vi "CheckLibraries.vi"(11 "hub":string) -> (0 "error out":errorcluster, 3 "console out":string)   [LabVIEW 2022 SP3]
panel:
  out "Array":bool[](array[boolean])
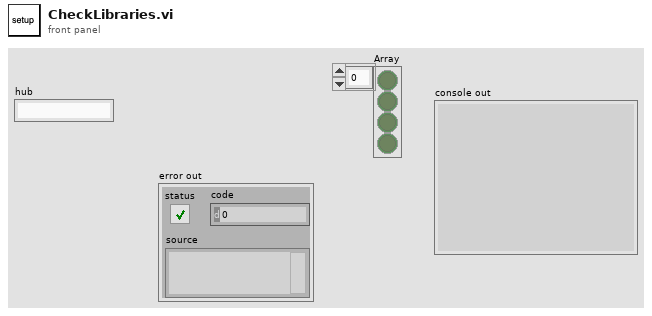
[diagram p1: front panel]
types:
  T1 = typedef "PythonCtrl.ctl" = cluster{"session":refnum<k35>, "PyPath":path, "Processor":T2, "Port":string, "version":string}
  T2 = typedef "Processors.ctl" = enum16{"SPIKE", "Pi", "Pi_ssh", "OpenMV", "Dunio"}
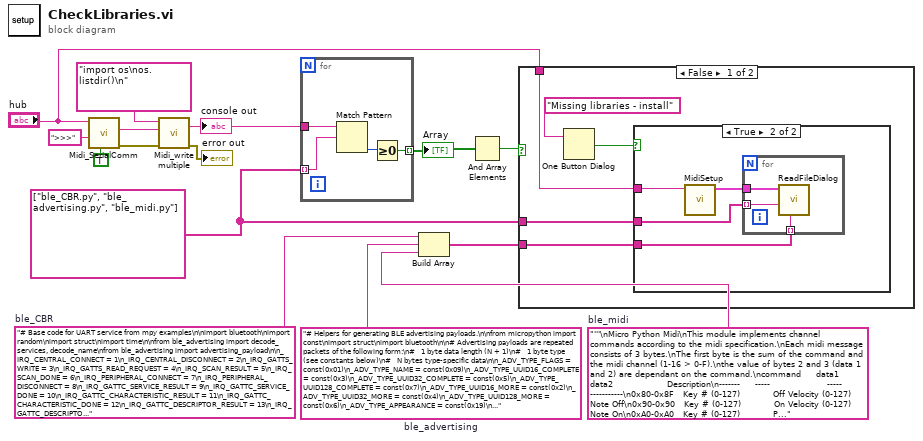
[diagram p0: block diagram]
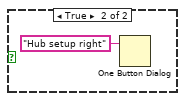
[diagram p3: hidden frame]
diagram:
  w4 = "'''\nMicro Python Midi\nThis module implements channel commands according to the midi specification.\nEach midi message consists of 3 bytes.\nThe first byte is the sum of the command and the midi channel (1-16 > 0-F).\nthe value of bytes 2 and 3 (data 1 and 2) are dependant on the command.\ncommand     data1                   data2                  Description\n-------     -----                   -----                  -----------\n0x80-0x8F   Key # (0-127)           Off Velocity (0-127)   Note Off\n0x90-0x90   Key # (0-127)           On Velocity (0-127)    Note On\n0xA0-0xA0   Key # (0-127)           Pressure (0-127)       Poly Pressure\n0xB0-0xB0   Control # (0-127)       Control Value (0-127)  Control\n0xC0-0xC0   Program # (0-127)       Not Used (send 0)      Program Change\n0xD0-0xD0   Pressure Value (0-127)  Not Used (send 0)      Channel Pressure\n0xE0-0xE0   Range LSB (0-127)       Range MSB (0-127)      Pitch Bend\nhttp://www.midi.org/techspecs/midimessages.php\n'''\n\nimport struct\nimport ble_CBR\nimport bluetooth\nimport button\nimport time\nimport distance_sensor as ds\nimport port,time\nimport color_sensor as cs\n\ndone = lambda : button.button_pressed(button.BUTTON_RIGHT)\n\npackage = [0x00,0x00,0x00,0x00,0x00]\n\nclass midi:\n    def __init__(self, name = 'MySpike'):\n        n = name[0:7]\n        self.connection = ble_CBR.BLESimplePeripheral(bluetooth.BLE(), 'MIDI', n)\n        self.connection.on_write(self.on_receive)\n        self.buffer = []\n        \n    def on_receive(self, msg):\n        print(\"RX: \", msg)\n      \n    def connected(self):\n        return self.connection.is_connected()\n\n    def convert(self, cmd, value, volume):\n        timestamp_ms = time.ticks_ms()\n        package[0] = (timestamp_ms >> 7 & 0b111111) | 0x80\n        package[1] =  0x80 | (timestamp_ms & 0b1111111)\n        package[2] =  0x80 | cmd\n        package[3] = value\n        package[4] = volume\n        return struct.pack(\"bbbbb\", package[0], package[1], package[2], package[3], package[4])\n\n    def NoteOn(self, note = 40, volume = 127):  \n        if self.connected():\n            self.connection.send(self.convert(0x90,note,volume))\n            self.buffer.insert(0,note)  # put in front\n        else:\n            print('not connected')\n            \n    def NoteOff(self, note = 40):\n        if self.connected():\n            self.connection.send(self.convert(0x80,note,0))\n            try:\n                self.buffer.remove(note)\n            except:\n                pass\n        \n    def NewNote(self, note = 40, volume = 127):\n        self.AllOff()\n        self.NoteOn(note,volume)\n        \n    def AllOff(self):\n        for note in self.buffer:\n            self.NoteOff(note) \n        \n    def test(self, duration = 1):\n        notes = [60,61,62,63,64,63,62,61]\n        for note in notes:\n            self.NewNote(note)\n            time.sleep(duration)\n        self.AllOff()\n        \n    def close(self):\n        self.AllOff()\n        self.connection.disconnect()\n    \n'''\np1 = port.PORTD\np2 = port.PORTF\nlight = port.PORTA\n    \nfred = midi('ChrisSPIKE')\n\nwhile not done:\n    d = ds.get_distance(p)\n    cs.get_color(light)]\n    cs.get_reflection(light)\n    if fred.connected():\n        fred.NewNote((d-40)/15+48)\nfred.close()\n'''"  # ble_midi
  w5 = "# Helpers for generating BLE advertising payloads.\n\nfrom micropython import const\nimport struct\nimport bluetooth\n\n# Advertising payloads are repeated packets of the following form:\n#   1 byte data length (N + 1)\n#   1 byte type (see constants below)\n#   N bytes type-specific data\n\n_ADV_TYPE_FLAGS = const(0x01)\n_ADV_TYPE_NAME = const(0x09)\n_ADV_TYPE_UUID16_COMPLETE = const(0x3)\n_ADV_TYPE_UUID32_COMPLETE = const(0x5)\n_ADV_TYPE_UUID128_COMPLETE = const(0x7)\n_ADV_TYPE_UUID16_MORE = const(0x2)\n_ADV_TYPE_UUID32_MORE = const(0x4)\n_ADV_TYPE_UUID128_MORE = const(0x6)\n_ADV_TYPE_APPEARANCE = const(0x19)\n\n\n# Generate a payload to be passed to gap_advertise(adv_data=...).\ndef advertising_payload(limited_disc=False, br_edr=False, name=None, services=None, appearance=0):\n    payload = bytearray()\n\n    def _append(adv_type, value):\n        nonlocal payload\n        payload += struct.pack(\"BB\", len(value) + 1, adv_type) + value\n\n    _append(_ADV_TYPE_FLAGS,struct.pack(\"B\", (0x01 if limited_disc else 0x02) + (0x18 if br_edr else 0x04)),)\n\n    if name:\n        _append(_ADV_TYPE_NAME, name)\n\n    if services:\n        for uuid in services:\n            b = bytes(uuid)\n            if len(b) == 2:\n                _append(_ADV_TYPE_UUID16_COMPLETE, b)\n            elif len(b) == 4:\n                _append(_ADV_TYPE_UUID32_COMPLETE, b)\n            elif len(b) == 16:\n                _append(_ADV_TYPE_UUID128_COMPLETE, b)\n\n    # See org.bluetooth.characteristic.gap.appearance.xml\n    if appearance:\n        _append(_ADV_TYPE_APPEARANCE, struct.pack(\"<h\", appearance))\n\n    return payload\n\n\ndef decode_field(payload, adv_type):\n    i = 0\n    result = []\n    while i + 1 < len(payload):\n        if payload[i + 1] == adv_type:\n            result.append(payload[i + 2 : i + payload[i] + 1])\n        i += 1 + payload[i]\n    return result\n\n\ndef decode_name(payload):\n    n = decode_field(payload, _ADV_TYPE_NAME)\n    return str(n[0], \"utf-8\") if n else \"\"\n\n\ndef decode_services(payload):\n    services = []\n    for u in decode_field(payload, _ADV_TYPE_UUID16_COMPLETE):\n        services.append(bluetooth.UUID(struct.unpack(\"<h\", u)[0]))\n    for u in decode_field(payload, _ADV_TYPE_UUID32_COMPLETE):\n        services.append(bluetooth.UUID(struct.unpack(\"<d\", u)[0]))\n    for u in decode_field(payload, _ADV_TYPE_UUID128_COMPLETE):\n        services.append(bluetooth.UUID(u))\n    return services\n\n\ndef demo():\n    payload = advertising_payload(name=\"mp2\",services=[bluetooth.UUID(0x181A), bluetooth.UUID(\"6E400001-B5A3-F393-E0A9-E50E24DCCA9E\")],)\n    print(payload)\n    print(decode_name(payload))\n    print(decode_services(payload))\n\n\nif __name__ == \"__main__\":\n    demo()\n"  # ble_advertising
  w6 = "# Base code for UART service from mpy examples\n\nimport bluetooth\nimport random\nimport struct\nimport time\n\nfrom ble_advertising import decode_services, decode_name\nfrom ble_advertising import advertising_payload\n\n_IRQ_CENTRAL_CONNECT = 1\n_IRQ_CENTRAL_DISCONNECT = 2\n_IRQ_GATTS_WRITE = 3\n_IRQ_GATTS_READ_REQUEST = 4\n_IRQ_SCAN_RESULT = 5\n_IRQ_SCAN_DONE = 6\n_IRQ_PERIPHERAL_CONNECT = 7\n_IRQ_PERIPHERAL_DISCONNECT = 8\n_IRQ_GATTC_SERVICE_RESULT = 9\n_IRQ_GATTC_SERVICE_DONE = 10\n_IRQ_GATTC_CHARACTERISTIC_RESULT = 11\n_IRQ_GATTC_CHARACTERISTIC_DONE = 12\n_IRQ_GATTC_DESCRIPTOR_RESULT = 13\n_IRQ_GATTC_DESCRIPTOR_DONE = 14\n_IRQ_GATTC_READ_RESULT = 15\n_IRQ_GATTC_READ_DONE = 16\n_IRQ_GATTC_WRITE_DONE = 17\n_IRQ_GATTC_NOTIFY = 18\n_IRQ_GATTC_INDICATE = 19\n\n_ADV_IND = 0x00\n_ADV_DIRECT_IND = 0x01\n_ADV_SCAN_IND = 0x02\n_ADV_NONCONN_IND = 0x03\n\n_UART_SERVICE_UUID = bluetooth.UUID(\"6E400001-B5A3-F393-E0A9-E50E24DCCA9E\")\n_UART_RX_CHAR_UUID = bluetooth.UUID(\"6E400002-B5A3-F393-E0A9-E50E24DCCA9E\")\n_UART_TX_CHAR_UUID = bluetooth.UUID(\"6E400003-B5A3-F393-E0A9-E50E24DCCA9E\")\n\n_FLAG_READ = 0x0002\n_FLAG_WRITE_NO_RESPONSE = 0x0004\n_FLAG_WRITE = 0x0008\n_FLAG_NOTIFY = 0x0010\n\n_UART_UUID = _UART_SERVICE_UUID\n_UART_TX = (_UART_TX_CHAR_UUID, _FLAG_READ | _FLAG_NOTIFY,)\n_UART_RX = (_UART_RX_CHAR_UUID, _FLAG_WRITE | _FLAG_WRITE_NO_RESPONSE,)\n_UART_SERVICE = (_UART_UUID,(_UART_TX, _UART_RX),)\n\n_MIDI_SERVICE_UUID = bluetooth.UUID(\"03B80E5A-EDE8-4B33-A751-6CE34EC4C700\")\n_MIDI_CHAR_UUID = bluetooth.UUID(\"7772E5DB-3868-4112-A1A9-F2669D106BF3\")\n\n_MIDI_UUID = _MIDI_SERVICE_UUID\n_MIDI_TXRX = (_MIDI_CHAR_UUID, _FLAG_READ | _FLAG_NOTIFY | _FLAG_WRITE_NO_RESPONSE,)\n_MIDI_SERVICE = (_MIDI_UUID,(_MIDI_TXRX,),)\n\n#------------------------------------Peripheral-------------------------------\n\nclass BLESimplePeripheral:\n    def __init__(self, ble, type = 'UART', name=\"SPIKE\"):\n        self.type = type\n        services = [_UART_UUID] if type == 'UART' else [_MIDI_UUID]\n        self._ble = ble\n        self._ble.active(True)\n        self._ble.irq(self._irq)\n        if self.type == 'UART':\n            ((self._handle_tx, self._handle_rx),) = self._ble.gatts_register_services((_UART_SERVICE,))\n            services = [_UART_UUID]\n            print('setup as uart')\n        else:\n            ((self._handle_tx, ),) = self._ble.gatts_register_services((_MIDI_SERVICE,))\n            self._handle_rx = self._handle_tx   # same handle for both directions\n            services = [_MIDI_UUID]\n            print('setup as midi')\n        self._connections = set()\n        self._write_callback = None\n        self._payload = advertising_payload(name=name, services=services)\n        self._advertise()\n\n    def _irq(self, event, data):\n        # Track connections so we can send notifications.\n        if event == _IRQ_CENTRAL_CONNECT:\n            conn_handle, _, _ = data\n            print(\"New connection\", conn_handle)\n            self._connections.add(conn_handle)\n        elif event == _IRQ_CENTRAL_DISCONNECT:\n            conn_handle, _, _ = data\n            print(\"Disconnected\", conn_handle)\n            self._connections.remove(conn_handle)\n            self._write_callback = None\n            # Start advertising again to allow a new connection.\n            #self._advertise()\n        elif event == _IRQ_GATTS_WRITE:\n            conn_handle, value_handle = data\n            value = self._ble.gatts_read(value_handle)\n            if value_handle == self._handle_rx and self._write_callback:\n                self._write_callback(value)\n\n    def send(self, data):\n        for conn_handle in self._connections:\n            self._ble.gatts_notify(conn_handle, self._handle_tx, data)\n\n    def is_connected(self):\n        return len(self._connections) > 0\n\n    def _advertise(self, interval_us=500000):\n        print(\"Starting advertising\")\n        self._ble.gap_advertise(interval_us, adv_data=self._payload)\n\n    def on_write(self, callback):\n        self._write_callback = callback\n        \n    def disconnect(self):\n        if not self._conn_handle:\n            return\n        self._ble.gap_disconnect(self._conn_handle)\n\n#------------------------------------Central-------------------------------\n\nclass BLESimpleCentral:     #only for UART - all midi is peripheral\n    def __init__(self, ble): \n        self._ble = ble\n        self._ble.active(True)\n        self._ble.irq(self._irq)\n\n        self._reset()\n\n    def _reset(self):\n        # Cached name and address from a successful scan.\n        self._name = None\n        self._addr_type = None\n        self._addr = None\n\n        # Callbacks for completion of various operations.\n        # These reset back to None after being invoked.\n        self._scan_callback = None\n        self._conn_callback = None\n        self._read_callback = None\n\n        # Persistent callback for when new data is notified from the device.\n        self._notify_callback = None\n\n        # Connected device.\n        self._conn_handle = None\n        self._start_handle = None\n        self._end_handle = None\n        self._tx_handle = None\n        self._rx_handle = None\n\n    def _irq(self, event, data):\n        if event == _IRQ_SCAN_RESULT:\n            addr_type, addr, adv_type, rssi, adv_data = data\n            if adv_type in (_ADV_IND, _ADV_DIRECT_IND) and _UART_SERVICE_UUID in decode_services(adv_data):\n                # Found a potential device, remember it and stop scanning.\n                self._addr_type = addr_type\n                self._addr = bytes(addr)  # Note: addr buffer is owned by caller so need to copy it.\n                self._name = decode_name(adv_data) or \"?\"\n                self._ble.gap_scan(None)\n\n        elif event == _IRQ_SCAN_DONE:\n            if self._scan_callback:\n                if self._addr:\n                    # Found a device during the scan (and the scan was explicitly stopped).\n                    self._scan_callback(self._addr_type, self._addr, self._name)\n                    self._scan_callback = None\n                else:\n                    # Scan timed out.\n                    self._scan_callback(None, None, None)\n\n        elif event == _IRQ_PERIPHERAL_CONNECT:\n            # Connect successful.\n            conn_handle, addr_type, addr = data\n            if addr_type == self._addr_type and addr == self._addr:\n                self._conn_handle = conn_handle\n                self._ble.gattc_discover_services(self._conn_handle)\n\n        elif event == _IRQ_PERIPHERAL_DISCONNECT:\n            # Disconnect (either initiated by us or the remote end).\n            conn_handle, _, _ = data\n            if conn_handle == self._conn_handle:\n                # If it was initiated by us, it'll already be reset.\n                self._reset()\n\n        elif event == _IRQ_GATTC_SERVICE_RESULT:\n            # Connected device returned a service.\n            conn_handle, start_handle, end_handle, uuid = data\n            print(\"service\", data)\n            if conn_handle == self._conn_handle and uuid == _UART_SERVICE_UUID:\n                self._start_handle, self._end_handle = start_handle, end_handle\n\n        elif event == _IRQ_GATTC_SERVICE_DONE:\n            # Service query complete.\n            if self._start_handle and self._end_handle:\n                self._ble.gattc_discover_characteristics(self._conn_handle, self._start_handle, self._end_handle)\n            else:\n                print(\"Failed to find uart service.\")\n\n        elif event == _IRQ_GATTC_CHARACTERISTIC_RESULT:\n            # Connected device returned a characteristic.\n            conn_handle, def_handle, value_handle, properties, uuid = data\n            if conn_handle == self._conn_handle and uuid == _UART_RX_CHAR_UUID:\n                self._rx_handle = value_handle\n            if conn_handle == self._conn_handle and uuid == _UART_TX_CHAR_UUID:\n                self._tx_handle = value_handle\n\n        elif event == _IRQ_GATTC_CHARACTERISTIC_DONE:\n            # Characteristic query complete.\n            if self._tx_handle is not None and self._rx_handle is not None:\n                # We've finished connecting and discovering device, fire the connect callback.\n                if self._conn_callback:\n                    self._conn_callback()\n            else:\n                print(\"Failed to find uart rx characteristic.\")\n\n        elif event == _IRQ_GATTC_WRITE_DONE:\n            conn_handle, value_handle, status = data\n            print(\"TX complete\")\n\n        elif event == _IRQ_GATTC_NOTIFY:\n            conn_handle, value_handle, notify_data = data\n            if conn_handle == self._conn_handle and value_handle == self._tx_handle:\n                if self._notify_callback:\n                    self._notify_callback(notify_data)\n\n    # Returns true if we've successfully connected and discovered characteristics.\n    def is_connected(self):\n        return (self._conn_handle is not None and self._tx_handle is not None and self._rx_handle is not None)\n\n    # Find a device advertising the environmental sensor service.\n    def scan(self, callback=None):\n        self._addr_type = None\n        self._addr = None\n        self._scan_callback = callback\n        self._ble.gap_scan(2000, 30000, 30000)\n\n    # Connect to the specified device (otherwise use cached address from a scan).\n    def connect(self, addr_type=None, addr=None, callback=None):\n        self._addr_type = addr_type or self._addr_type\n        self._addr = addr or self._addr\n        self._conn_callback = callback\n        if self._addr_type is None or self._addr is None:\n            return False\n        self._ble.gap_connect(self._addr_type, self._addr)\n        return True\n\n    # Disconnect from current device.\n    def disconnect(self):\n        if not self._conn_handle:\n            return\n        self._ble.gap_disconnect(self._conn_handle)\n        self._reset()\n\n    # Send data over the UART\n    def write(self, v, response=False):\n        if not self.is_connected():\n            return\n        self._ble.gattc_write(self._conn_handle, self._rx_handle, v, 1 if response else 0)\n\n    # Set handler for when data is received over the UART.\n    def on_notify(self, callback):\n        self._notify_callback = callback\n"  # ble_CBR
  w3 = string[] ["ble_CBR.py", "ble_advertising.py", "ble_midi.py"]
  n1 = call "Midi_SerialComm.vi"("CtrlC"=TRUE, "wait for"=">>>", "hub"="hub") -> ("error out"=w14:errorcluster, "read"=w13:string)  [unwired: 7 in]
  n2 = call "Midi_write multiple.vi"("error in (no error)"=w14, "console in"=w13, "to write"="import os\nos.listdir()\n") -> ("error out"=→"error out":errorcluster, "console out"=w9:string)  [unwired: 7 in]
  "console out" <- w9
  n3 = for {
    tunnel: w9 -> [w19]
    tunnel: w3 -> [w18] mode=indexing
    tunnel: [w16] -> w8 mode=indexing
    n4 = Match Pattern(string=w19, regular expression=w18) -> (offset past match=w17:i32)  [unwired: 1 in, 3 out]
    n5 = Greater Or Equal To 0?(x=w17) -> (x >= 0?=w16:bool)
  }
  "Array" <- w8
  n6 = Build Array(w6, w5, w4) -> (w2:string[])
  n7 = And Array Elements(Boolean array=w8) -> (logical AND=w7:bool)
  n8 = case shown="False" w7 {
    tunnel: w3 -> [w23 _]
    tunnel: w2 -> [w22 _]
    tunnel: "hub" -> [w20 _]
    frame False {
      n9 = One Button Dialog(message="Missing libraries - install") -> (true=w21:bool)  [unwired: 1 in]
      n10 = case shown="True" w21 {
        tunnel: w23 -> [_ w27]
        tunnel: w22 -> [_ w26]
        tunnel: w20 -> [_ w25]
        frame False {
        }
        frame True {
          n11 = call "MidiSetup.vi"("hub"=w25) -> ("Python"=w28:T1)  [unwired: 8 in, 2 out]
          n12 = for {
            tunnel: w28 -> [w31]
            tunnel: w27 -> [w30] mode=indexing
            tunnel: w26 -> [w29] mode=indexing
            n13 = call "ReadFileDialog.vi"("File Text"=w29, "File name"=w30, "Python in"=w31) -> ()  [unwired: 7 in, 2 out]
          }
        }
      }
    }
    frame True {
      n14 = One Button Dialog(message="Hub setup right") -> ()  [unwired: 1 in, 1 out]
    }
  }
